vi "振动demo.vi"() -> ()   [LabVIEW 2020]
uses:
  Database/Global2.vi
  Global_Variable/Global.vi
  Global_Variable/Global1.vi
  Global_Variable/A131258.vi
  <vilib>/addons/database/Connection.llb/DB Tools Open Connec (String).vi
  <vilib>/addons/database/Connection.llb/Conn Execute.vi
  <vilib>/addons/database/Recordset.llb/Rec Fetch Recordset Data (R).vi
  <vilib>/Utility/config.llb/NI_LVConfig.lvlib
  <vilib>/addons/database/NI_Database_API.lvlib
panel:
  out "result":string
  out "FdeviceID":string
  out "deviceID":string
  out "USERID":string
  out "productID":string
  out "CODEID":string
  in  "附加信息":string
  in  "设备状态":enum16{"设备离线", "设备正常", "设备缺料", "设备故障", "质量报警"}(ring)=enum."设备故障"
  in  "附加信息 2":string
  in  "设备状态 2":enum16{"设备离线", "设备正常", "设备缺料", "设备故障", "质量报警"}(ring)=enum."设备缺料"
  in  "附加信息 3":string
  in  "设备状态 3":enum16{"设备离线", "设备正常", "设备缺料", "设备故障", "质量报警"}(ring)=enum."质量报警"
  out "产品型号":string
  out "联机模式":string
  out "用户权限":string
  out "用户名":string
  in  "判定结果1":bool[][](array[boolean])=[[TRUE]]
  in  "选项卡控件 2":enum32{"主页面", "参数设置"}(tab)
  out "产品条码":string
  out "判定结果":bool
  out "振动NHV-FFT":cluster{"f0":dbl, "df":dbl, "magnitude":dbl[]}[](graph)
  out "振动NVH-Order":cluster{"f0":dbl, "df":dbl, "magnitude":dbl[]}[](graph)
  in  "表格控件":string[][](table)
  in  "设备故障":bool
  in  "设备缺料":bool
  in  "质量报警":bool
  out "上序结果":bool
  out "字符串":string
  in  "请输入添加的产品名称":string
  in  "请选择要删除的产品":string(combo)
  in  "振动判定范围":T1={"频率检测段1范围"={"单位"="Hz", "下限"=0.0, "上限"=100.0}, "频率检测段2范围"={"单位"="Hz", "下限"=100.0, "上限"=1000.0}, "频率检测段3范围"={"单位"="Hz", "下限"=1000.0, "上限"=2000.0}, "频率检测段4范围"={"单位"="Hz", "下限"=2000.0, "上限"=3000.0}, "频率检测段5范围"={"单位"="Hz", "下限"=3000.0, "上限"=10000.0}}
  in  "振动判定":T2={"频率检测段1振幅"={"单位"="dB", "下限"=0.0, "上限"=50.0}, "频率检测段2振幅"={"单位"="dB", "下限"=0.0, "上限"=40.0}, "频率检测段3振幅"={"单位"="dB", "下限"=0.0, "上限"=40.0}, "频率检测段4振幅"={"单位"="dB", "下限"=0.0, "上限"=40.0}, "频率检测段5振幅"={"单位"="dB", "下限"=0.0, "上限"=40.0}}
  in  "产品型号":string(combo)
  in  "删除":bool
  in  "确定":bool
  in  "添加":bool
  in  "退出":bool
  in  "更新":bool
  in  "确定按钮":bool
  # "060芯轴总成NVH评价"
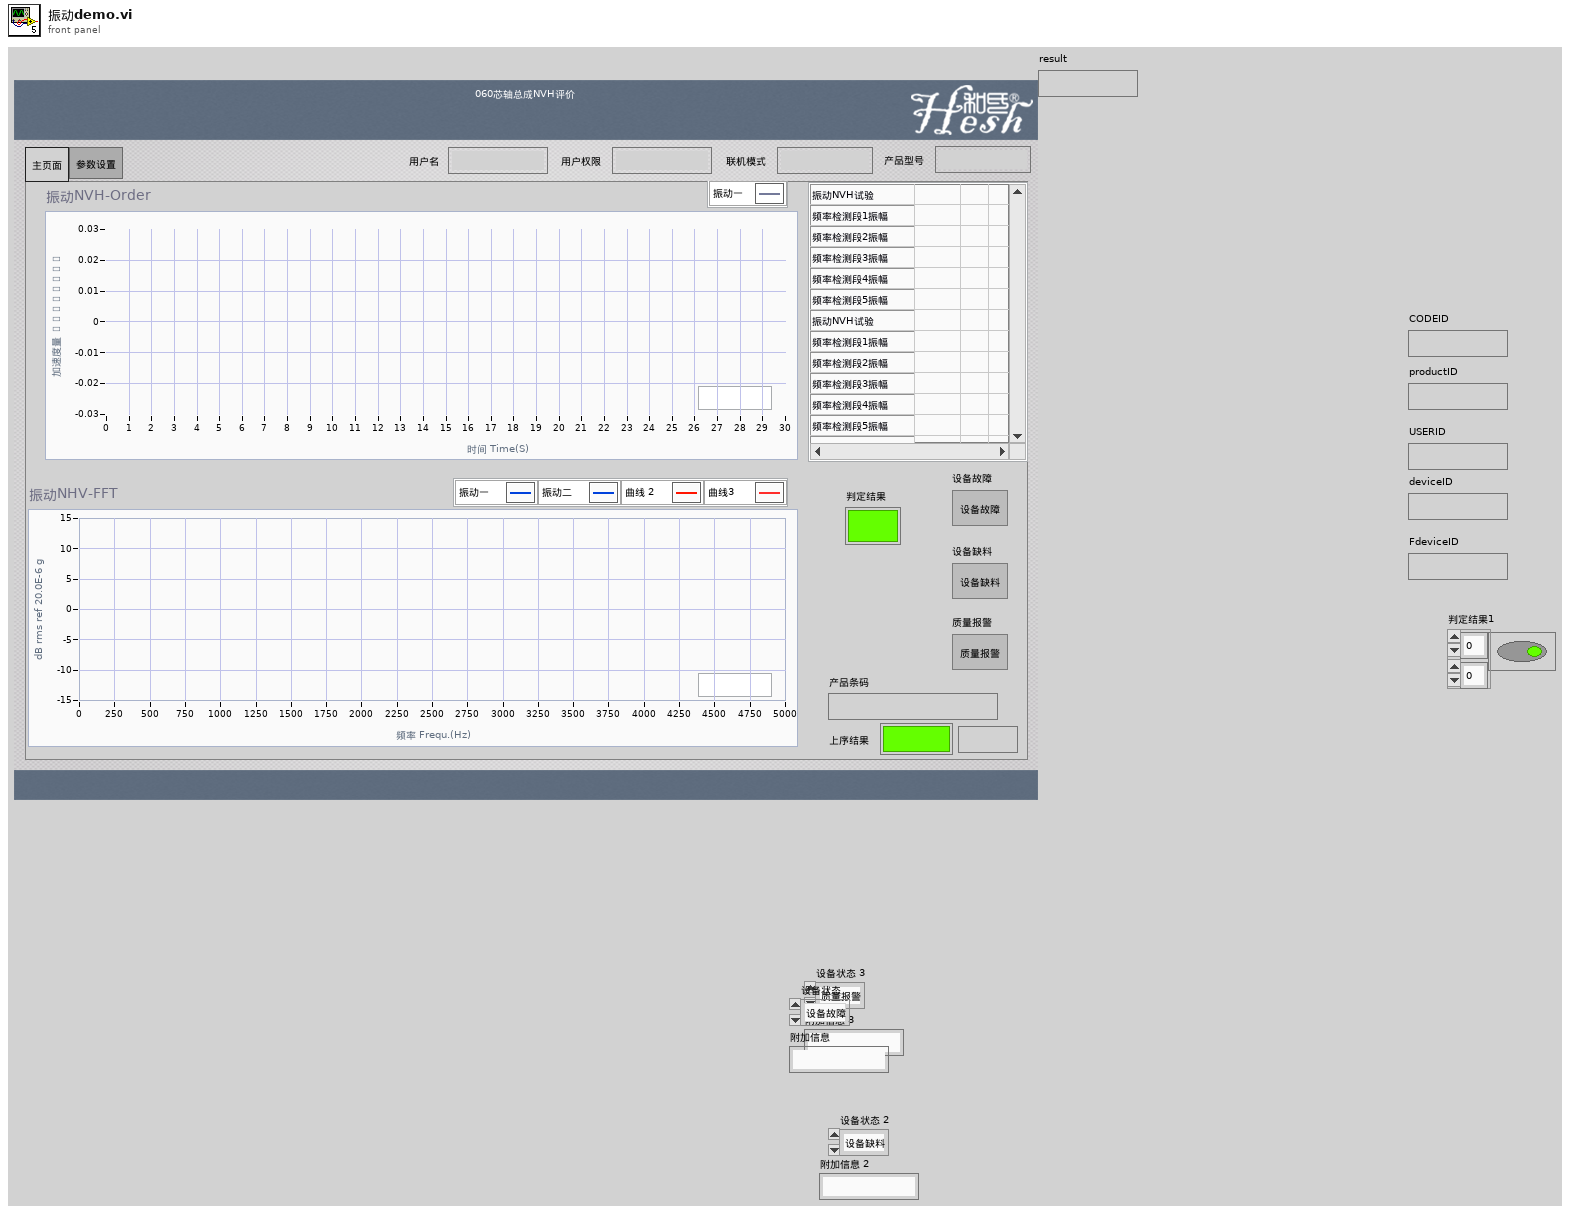
[diagram p1: front panel]
types:
  T1 = cluster{"频率检测段1范围":cluster{"单位":string, "下限":dbl, "上限":dbl}, "频率检测段2范围":cluster{"单位":string, "下限":dbl, "上限":dbl}, "频率检测段3范围":cluster{"单位":string, "下限":dbl, "上限":dbl}, "频率检测段4范围":cluster{"单位":string, "下限":dbl, "上限":dbl}, "频率检测段5范围":cluster{"单位":string, "下限":dbl, "上限":dbl}}
  T2 = cluster{"频率检测段1振幅":cluster{"单位":string, "下限":dbl, "上限":dbl}, "频率检测段2振幅":cluster{"单位":string, "下限":dbl, "上限":dbl}, "频率检测段3振幅":cluster{"单位":string, "下限":dbl, "上限":dbl}, "频率检测段4振幅":cluster{"单位":string, "下限":dbl, "上限":dbl}, "频率检测段5振幅":cluster{"单位":string, "下限":dbl, "上限":dbl}}
  T3 = cluster{"设备名称":string, "操作人员":string, "设备状态":enum16{"设备离线", "设备正常", "设备缺料", "设备故障", "质量报警"}, "附加信息":string}
  T4 = enum32{"Invalid", "Standard", "Closed", "Hidden", "Minimized", "Maximized"}
  T5 = cluster{"用户编号":string, "用户名":string, "用户密码(密文)":string, "用户权限":string}
  T6 = typedef "svc_Spectrum Info.ctl" = cluster{"channel name":string, "description":string, "x-axis units":T7, "spectral info":cluster{"spectrum type":T8, "linear/dB":enum16{"linear", "dB"}, "window":u16, "window size":i32, "FFT size":i32}, "engineering units":T9, "custom label":string, "dB reference [EU]":dbl, "peak units":enum16{"rms", "peak", "peak-peak"}, "weighting filter":T10, "spectral density?":bool, "unit label":string, "spectrum skewed?":bool, "complimentary spectrum units":T11}
  T7 = typedef "svc_X-Axis Units.ctl" = u16
  T8 = typedef "svc_Spectrum Type.ctl" = enum16{"FFT Spectrum [complex]", "Amplitude [Magnitude]", "Power [Magnitude^2]", "Cross Spectrum [complex]", "Frequency Response [Complex]"}
  T9 = typedef "svc_Engineering Units Text Ring.ctl" = u16
  T10 = typedef "svc_Weighting Filter Text Ring.ctl" = u16
  T11 = typedef "svc_Complimentary Spectrum Units.ctl" = enum16{"none", "radians", "degrees", "cycles", "imaginary"}
  T12 = cluster{i64, i64, i64, "result":string, "result string":string}
  T13 = cluster{i64, i64, i64, "result":string, "result string":string}[]
  T14 = typedef "NI_Database_API.lvlib/Conn ObjectReference.ctl" = refnum<k1>
  T15 = cluster{i64, i64, "condition":string, dbl, "下限":dbl, "上限":dbl, string, string}
  T16 = cluster{i64, i64, "condition":string, dbl, "下限":dbl, "上限":dbl, string, string}[]
  T17 = cluster{i64, i64, dbl, "下限":dbl, "上限":dbl, string, string}
  T18 = typedef "NI_Database_API.lvlib/Rec ObjectReference.ctl" = refnum<k1>
  T19 = typedef "NI_LVConfig.lvlib/Config Data RefNum.ctl" = refnum<k1>
  T20 = cluster{"设备名称":string, "用户名":string, "设备状态":enum16{"设备离线", "设备正常", "设备缺料", "设备故障", "质量报警"}, "附加信息":string}
  T21 = cluster{"设备名称":string, "用户名":string, "设备状态 2":enum16{"设备离线", "设备正常", "设备缺料", "设备故障", "质量报警"}, "附加信息 2":string}
  T22 = cluster{"设备名称":string, "用户名":string, "设备状态 3":enum16{"设备离线", "设备正常", "设备缺料", "设备故障", "质量报警"}, "附加信息 3":string}
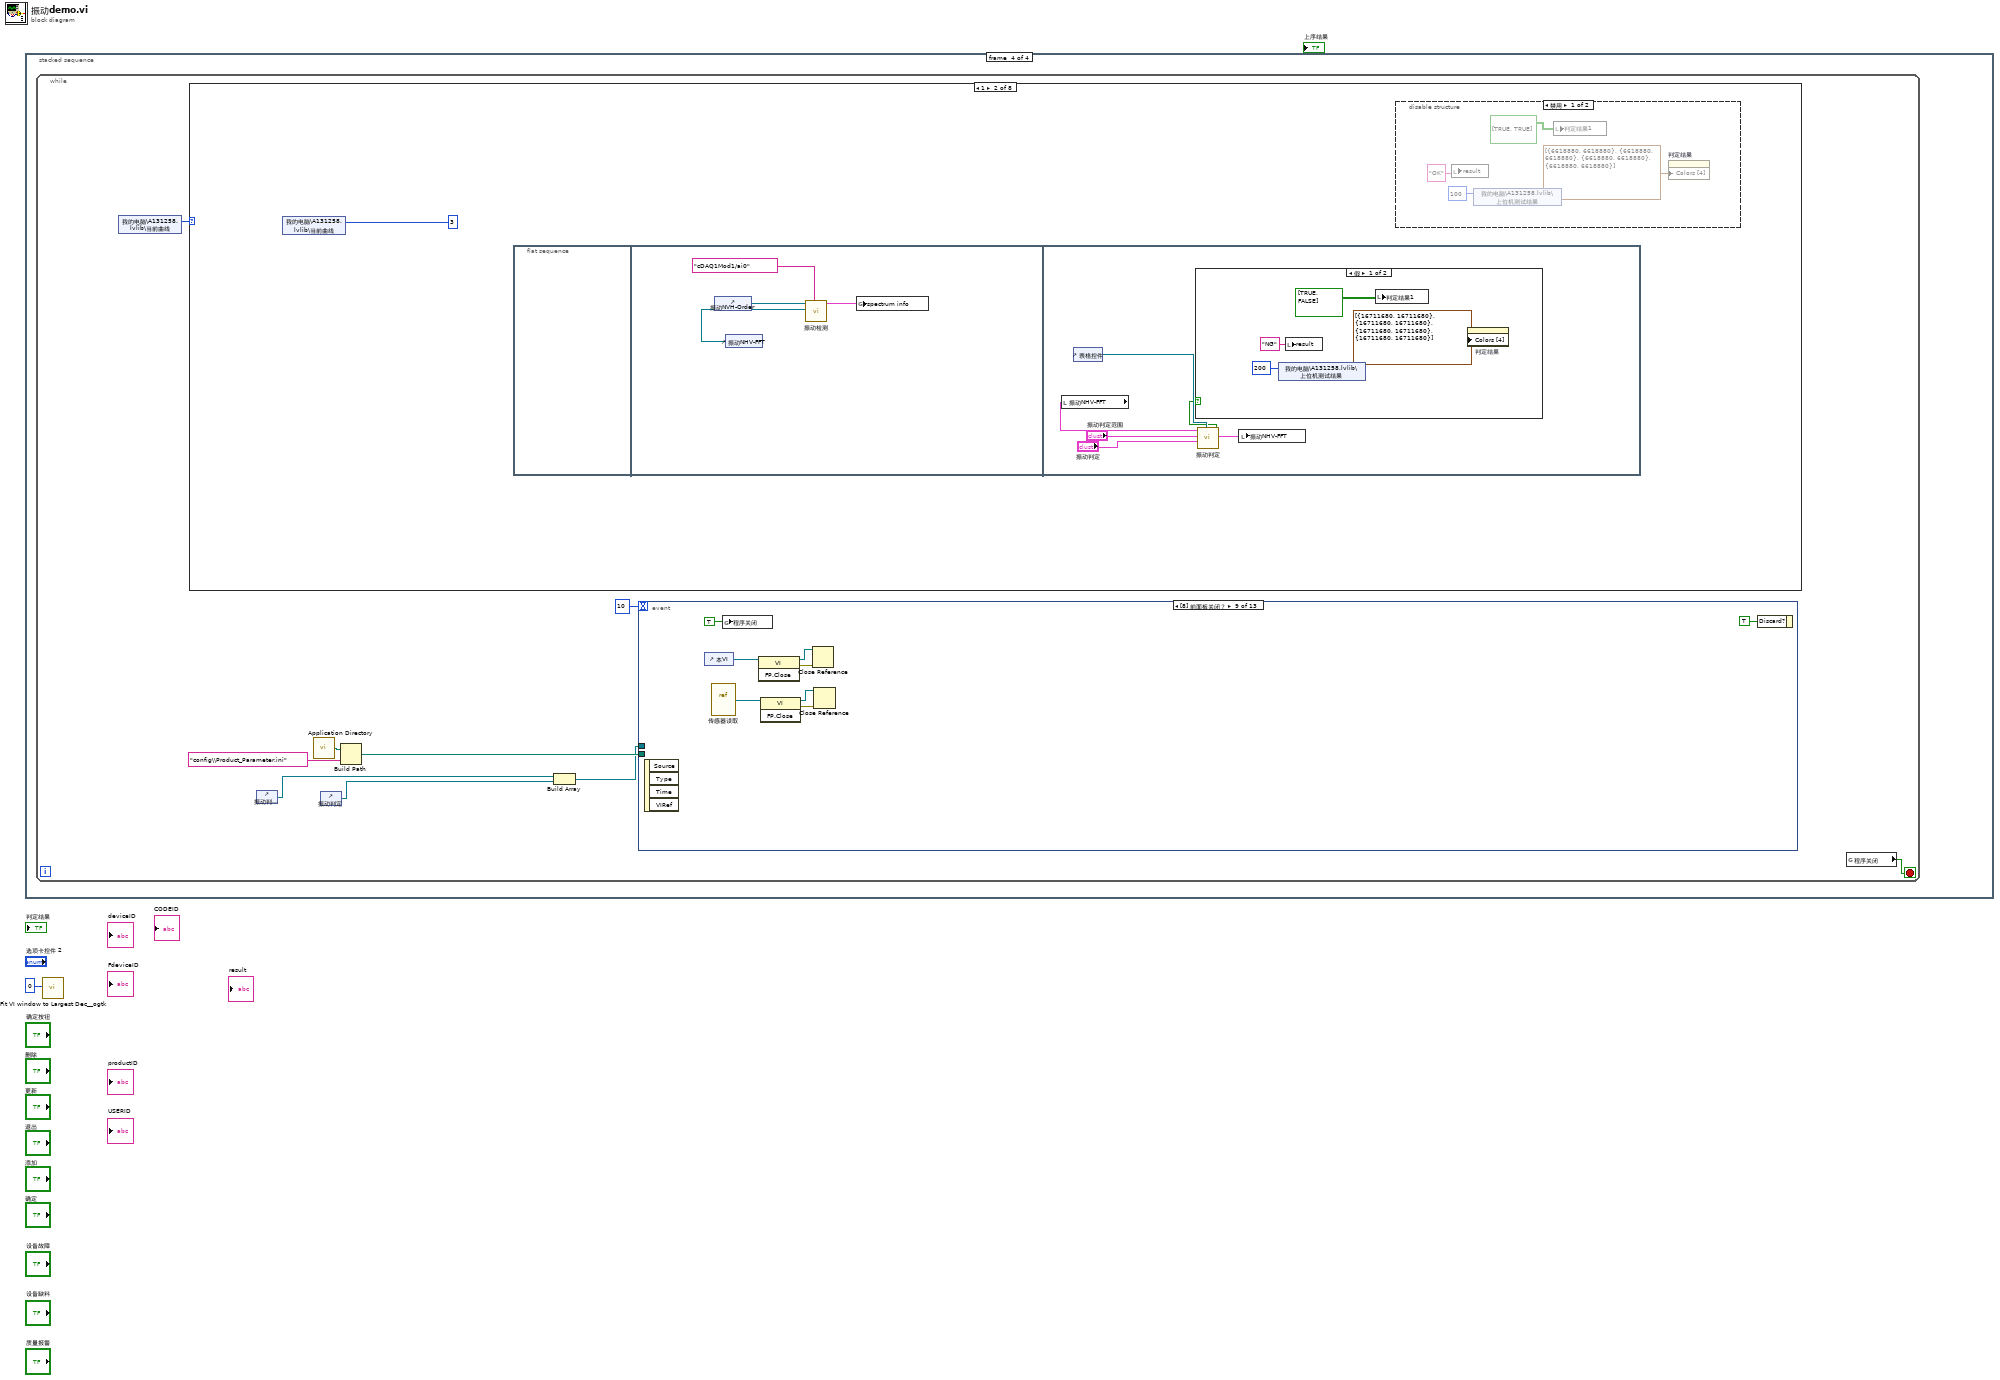
[diagram p0: block diagram]
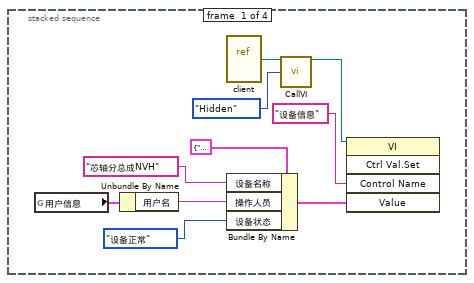
[diagram p2: hidden frame]
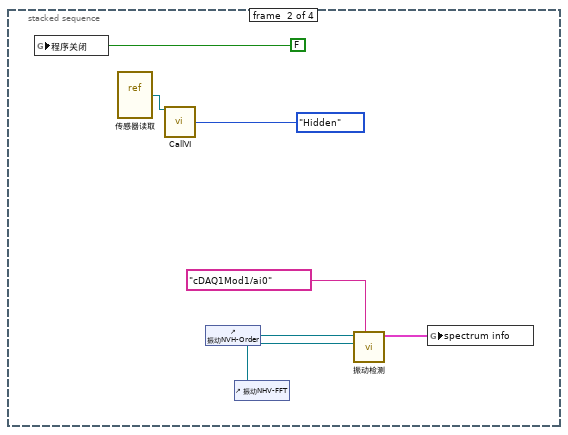
[diagram p3: hidden frame]
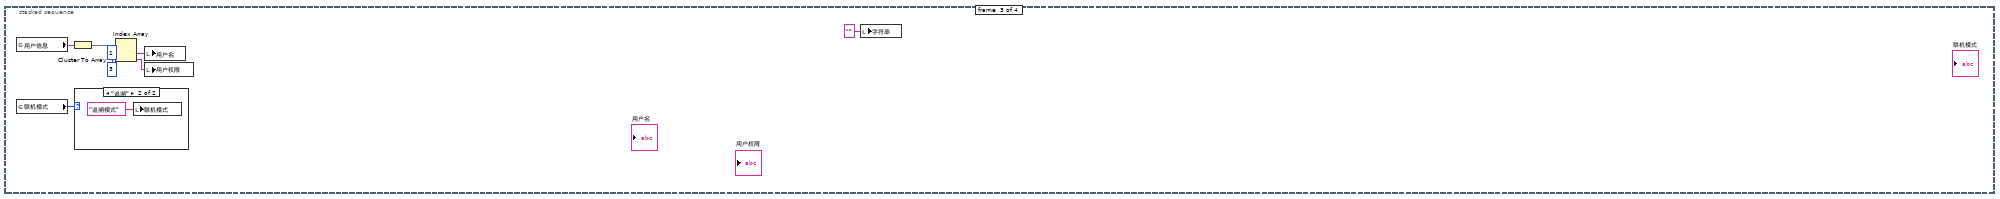
[diagram p4: hidden frame]
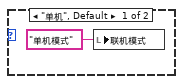
[diagram p5: hidden frame]
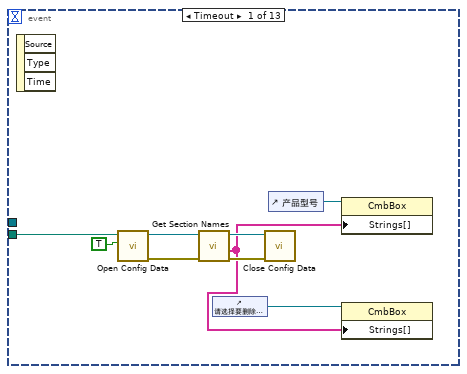
[diagram p6: hidden frame]
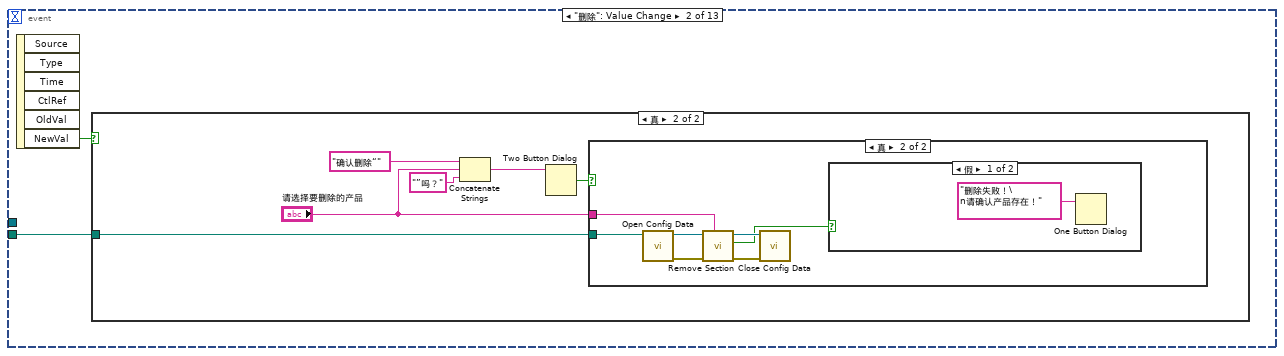
[diagram p7: hidden frame]
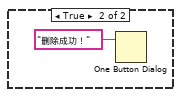
[diagram p10: hidden frame]
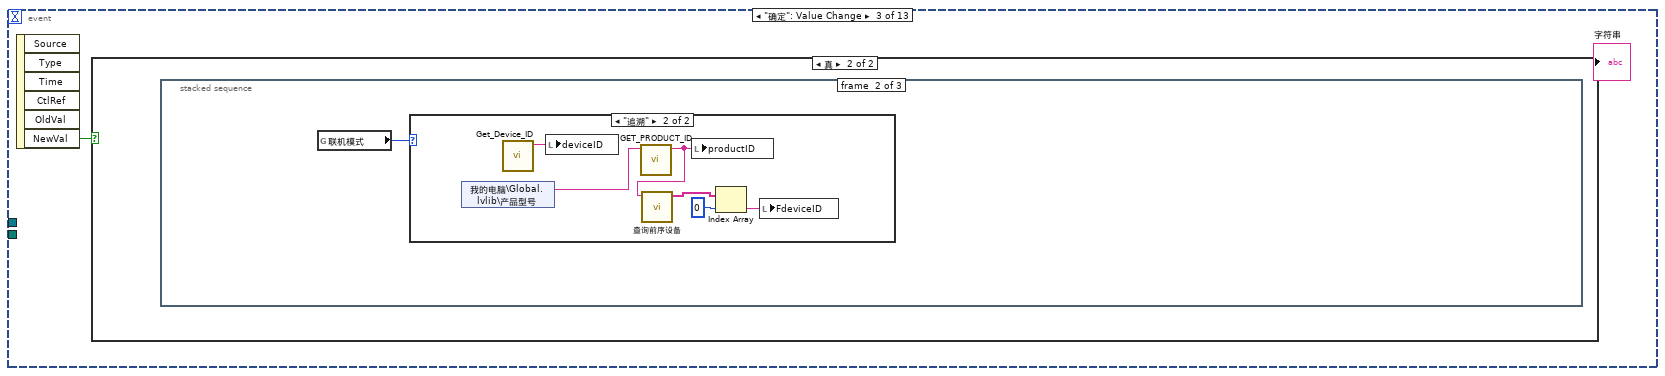
[diagram p11: hidden frame]
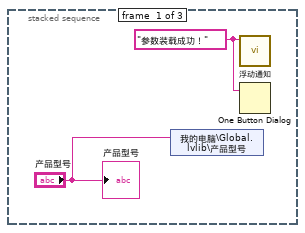
[diagram p13: hidden frame]
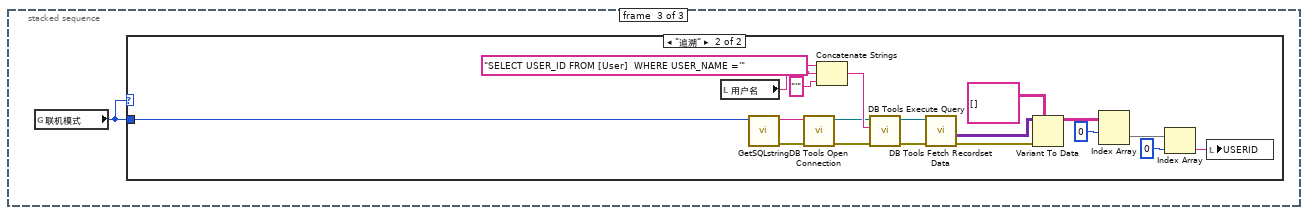
[diagram p15: hidden frame]
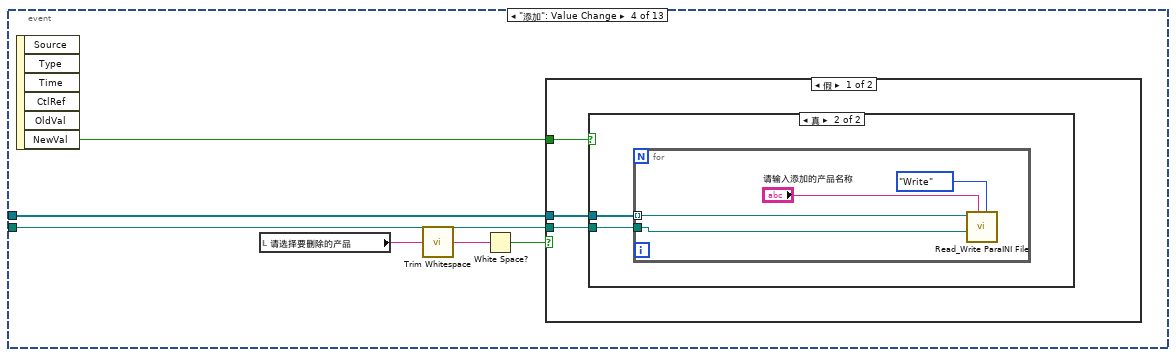
[diagram p17: hidden frame]
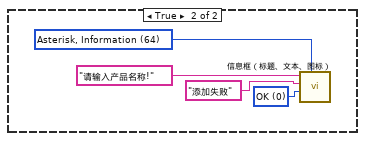
[diagram p19: hidden frame]
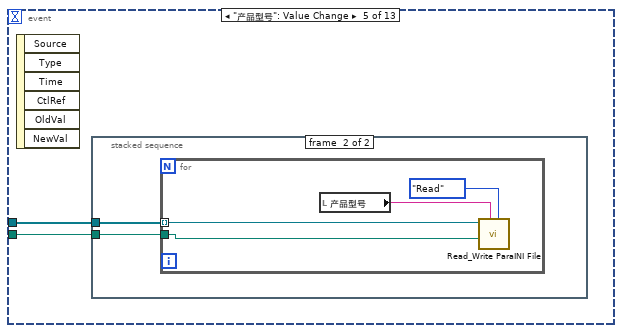
[diagram p20: hidden frame]
diagram:
  n1 = stacked-sequence {
    frame #0 {
      n2 = global read "Global2.vi" "用户信息"() -> (w11:T5)
      n3 = Unbundle By Name(w11) -> ("用户名"=w10:string)
      n4 = vi-ref "client.vi"() -> (w8:refnum<vi>)
      n5 = Bundle By Name(cluster=T3 {"设备名称"="", "操作人员"="", "设备状态"=enum."设备正常", "附加信息"=""} ("设备信息"), "设备名称"="芯轴分总成NVH", "操作人员"=w10, "设备状态"=enum16{"设备离线", "设备正常", "设备缺料", "设备故障", "质量报警"}."设备正常") -> (w9:T3)
      n6 = call "CallVI.vi"("VI引用"=w8, "状态"=T4."Hidden") -> ("VI引用输出"=w7:refnum<vi>)  [unwired: 11 in, 2 out]
      n7 = invoke class="VI" method="Ctrl Val.Set"(reference=w7, "Control Name"="设备信息" ("控件名"), "Value"=w9) -> ()  [unwired: 2 in, 5 out]
    }
    frame #1 {
      n8 = global write "Global.vi" "程序关闭"(FALSE ("程序关闭")) -> ()
      n9 = vi-ref "传感器读取.vi"() -> (w17:refnum<vi>)
      n10 = call "CallVI.vi"("VI引用"=w17, "状态"=T4."Hidden") -> ()  [unwired: 11 in, 3 out]
      n11 = control-ref of="振动NVH-Order"() -> (w15:refnum<vi>)
      n12 = control-ref of="振动NHV-FFT"() -> (w14:refnum<vi>)
      n13 = call "振动检测.vi"("通道输入"=tag "cDAQ1Mod1/ai0" ("DAQmx物理通道"), "WFGraph引用句柄FFT"=w14, "WFGraph引用句柄Order"=w15) -> ("spectrum info"=w13:T6[])  [unwired: 7 in, 1 out]
      n14 = global write "Global1.vi" "spectrum info"(w13) -> ()
    }
    frame #2 {
      n15 = global read "Global2.vi" "用户信息"() -> (w26:T5)
      n16 = global read "Global2.vi" "联机模式"() -> (w20:enum16{"单机", "追溯"})
      n17 = Cluster To Array(cluster=w26) -> (array=w25:string[])
      n18 = case shown="\"追溯\"" w20 {
        frame "单机", Default {
          n19 = local write "联机模式"("单机模式" ("联机模式")) -> ()
        }
        frame "追溯" {
          n20 = local write "联机模式"("追溯模式" ("联机模式")) -> ()
        }
      }
      n21 = Index Array(array=w25, index #1=1 ("索引"), index #2=3 ("索引")) -> (element #1=w22:string, element #2=w21:string)
      n22 = local write "用户名"(w22) -> ()
      n23 = local write "用户权限"(w21) -> ()
      n24 = local write "字符串"("" ("字符串")) -> ()
    }
    frame #3 {
      n25 = while {
        stop <- w29 stop-if-true
        n26 = shared-variable "我的电脑\\A131258.lvlib\\当前曲线"() -> (w37:i16)  [unwired: 1 in, 1 out]
        n27 = case shown="1" w37 {
          frame 0, Default {
          }
          frame 1 {
            n28 = shared-variable "我的电脑\\A131258.lvlib\\当前曲线"(i16 3 ("当前曲线")) -> ()  [unwired: 1 in, 1 out]
            n29 = flat-sequence {
              frame #0 {
              }
              frame #1 {
                n30 = control-ref of="振动NVH-Order"() -> (w194:refnum<vi>)
                n31 = control-ref of="振动NHV-FFT"() -> (w193:refnum<vi>)
                n32 = call "振动检测.vi"("通道输入"=tag "cDAQ1Mod1/ai0" ("DAQmx物理通道"), "WFGraph引用句柄FFT"=w193, "WFGraph引用句柄Order"=w194) -> ("spectrum info"=w191:T6[])  [unwired: 7 in, 1 out]
                n33 = global write "Global1.vi" "spectrum info"(w191) -> ()
              }
              frame #2 {
                n34 = local read "振动NHV-FFT"() -> (w200:cluster{"f0":dbl, "df":dbl, "magnitude":dbl[]}[])
                n35 = control-ref of="表格控件"() -> (w196:refnum<vi>)
                n36 = call "振动判定.vi"("Result"=w196, "振动判定"="振动判定", "振动判定范围"="振动判定范围", "FFT"=w200) -> ("FFT 2"=w197:cluster{"f0":dbl, "df":dbl, "magnitude":dbl[]}[], "OK？"=w195:bool)  [unwired: 6 in]
                n37 = case shown="假" w195 {
                  frame False {
                    n38 = shared-variable "我的电脑\\A131258.lvlib\\上位机测试结果"(i16 200 ("当前曲线")) -> ()  [unwired: 1 in, 1 out]
                    n39 = local write "result"("NG" ("result")) -> ()
                    n40 = local write "判定结果1"(bool[][] [[TRUE, FALSE]] ("判定结果1")) -> ()
                    n41 = property on="判定结果" class="Bool (严格)"("Colors [4]"=cluster{u32, u32}[] [{16711680, 16711680}, {16711680, 16711680}, {16711680, 16711680}, {16711680, 16711680}]) -> ()  [unwired: 2 in, 2 out]
                  }
                  frame True {
                    n42 = local write "result"("OK" ("result")) -> ()
                    n43 = shared-variable "我的电脑\\A131258.lvlib\\上位机测试结果"(i16 100 ("当前曲线")) -> ()  [unwired: 1 in, 1 out]
                    n44 = local write "判定结果1"(bool[][] [[TRUE, TRUE]] ("判定结果1")) -> ()
                    n45 = property on="判定结果" class="Bool (严格)"("Colors [4]"=cluster{u32, u32}[] [{6618880, 6618880}, {6618880, 6618880}, {6618880, 6618880}, {6618880, 6618880}]) -> ()  [unwired: 2 in, 2 out]
                  }
                }
                n46 = local write "振动NHV-FFT"(w197) -> ()
              }
            }
            n47 = disable-structure shown="禁用" {
              frame Disabled {
                n48 = local write "result"("OK" ("result")) -> ()
                n49 = shared-variable "我的电脑\\A131258.lvlib\\上位机测试结果"(i16 100 ("当前曲线")) -> ()  [unwired: 1 in, 1 out]
                n50 = local write "判定结果1"(bool[][] [[TRUE, TRUE]] ("判定结果1")) -> ()
                n51 = property on="判定结果" class="Bool (严格)"("Colors [4]"=cluster{u32, u32}[] [{6618880, 6618880}, {6618880, 6618880}, {6618880, 6618880}, {6618880, 6618880}]) -> ()  [unwired: 2 in, 2 out]
              }
              frame Enabled {
              }
            }
          }
          frame 2 {
            n52 = for {
              N: 6 -> [_]
              tunnel: [cluster{"f0":dbl, "df":dbl, "magnitude":dbl[]} {"f0"=0.0, "df"=0.0, "magnitude"=[]} ("power spectrum [dB EU]")] -> w212 mode=indexing
            }
            "振动NVH-Order" <- w212
            "振动NHV-FFT" <- w212
            n53 = property on="表格控件" class="Tbl (严格)"("Value"=string[][] [] ("表格控件"), "Row Headers[]"=string[] [] ("行首字符串[]")) -> ()  [unwired: 2 in, 2 out]
          }
          frame 3 {
            n54 = control-ref of="表格控件"() -> (w215:refnum<vi>)
            n55 = shared-variable "我的电脑\\A131258.lvlib\\当前曲线"(i16 4 ("当前曲线")) -> ()  [unwired: 1 in, 1 out]
            n56 = Wait (ms)(milliseconds to wait=u32 200 ("等待时间（毫秒）")) -> ()  [unwired: 1 out]
            n57 = control-ref of="振动NHV-FFT"() -> (w216:refnum<vi>)
            n58 = global write "Global.vi" "Result"(w215) -> ()
            n59 = control-ref of="振动NVH-Order"() -> (w214:refnum<vi>)
            n60 = global write "A131258.vi" "加速度"(w216) -> ()
            n61 = call "浮动通知.vi"("通知内容"="报表生成中") -> ()  [unwired: 11 in]
            n62 = global write "A131258.vi" "频率"(w214) -> ()
          }
          frame 4 {
            n63 = stacked-sequence {
              frame #0 {
                n64 = local read "产品条码"() -> (w220:string)
                n65 = call "Report_A131258.vi"("文件重命名"=TRUE, "文件名称"=w220, "布尔数组"="判定结果1") -> ()  [unwired: 8 in, 1 out]
              }
              frame #1 {
                n66 = global read "Global2.vi" "联机模式"() -> (w223:enum16{"单机", "追溯"})
                n67 = case shown="\"追溯\"" w223 {
                  frame "单机", Default {
                  }
                  frame "追溯" {
                    n68 = local read "result"() -> (w224:string)
                    n69 = local read "USERID"() -> (w250:string)
                    n70 = Decimal String To Number(string=w250, default (0L)=i64 0 ("默认(0 I32)")) -> (number=w251:i64)  [unwired: 1 in, 1 out]
                    n71 = local read "deviceID"() -> (w242:string)
                    n72 = global read "Global2.vi" "联机模式"() -> (w225:enum16{"单机", "追溯"})
                    n73 = local read "CODEID"() -> (w244:string)
                    n74 = Get Date/Time String(date format (0)=enum16{"short", "long", "abbreviated"}."short" ("日期格式(0)"), want seconds? (F)=FALSE ("需要秒？(F)")) -> (date string=w246:string, time string=w247:string)  [unwired: 1 in]
                    n75 = Decimal String To Number(string=w242, default (0L)=i64 0 ("默认(0 I32)")) -> (number=w243:i64)  [unwired: 1 in, 1 out]
                    n76 = Concatenate Strings(w246, " " ("字符串"), w247) -> (w249:string)
                    n77 = Decimal String To Number(string=w244, default (0L)=i64 0 ("默认(0 I32)")) -> (number=w245:i64)  [unwired: 1 in, 1 out]
                    n78 = Search and Replace String(replace all?=TRUE ("替换全部？(F)"), input string=w249, search string="/" ("替换字符串(\"\")"), replace string="-" ("替换字符串(\"\")")) -> (result string=w248:string)  [unwired: 4 in, 3 out]
                    n79 = Bundle(w243, w251, w245, "result"=w224, "result string"=w248) -> (w240:T12)  [unwired: 1 in]
                    n80 = call "GetSQLstring.vi"("联机模式"=w225) -> ("错误输出"=w237:errorcluster, "连接字符串"=w236:string)  [unwired: 9 in]
                    n81 = Build Array(w240) -> (w241:T13)
                    n82 = call-poly <vilib>:"DB Tools Open Connection.vi"("error in (no error)"=w237, "connection information"=w236) -> ("error out"=w235:errorcluster, "connection reference"=w238:T14)  [unwired: 6 in]
                    n83 = for {
                      tunnel: w241 -> [w256] mode=indexing
                      tunnel: w238 -> [w254]
                      shift-right: [w252] -> w239
                      shift-left: w235 -> [w259]
                      w255 = string[] ["DEVICE_ID", "USER_ID", "CODE_ID", "RESULT_VALUE", "RESULT_TIME"] ("columns")
                      w257 = "Result" ("table")
                      n84 = call <vilib>:"DB Tools Insert Data.vi"("data"=w256, "error in (no error)"=w259, "columns"=w255, "table"=w257, "connection reference"=w254) -> ("error out"=w258:errorcluster, "connection reference out"=w253:T14)  [unwired: 5 in]
                      n85 = case shown="错误" w258 {
                        selector: w258 -> [w260 w281]
                        tunnel: w255 -> [_ w278]
                        tunnel: w253 -> [w261 w270]
                        tunnel: w257 -> [_ w282]
                        tunnel: w256 -> [_ w274]
                        tunnel: [w261 w269] -> _
                        tunnel: [w260 w268] -> w252
                        frame No Error {
                        }
                        frame Error {
                          n86 = Array Subset(array=w278, index=3 ("长度"), length=2 ("长度")) -> (w279:string[])
                          n87 = Unbundle(w274) -> (w263:i64, w266:i64, "result"=w273:string, "result string"=w272:string)  [unwired: 1 out]
                          n88 = Bundle("result"=w273, "result string"=w272) -> (w271:cluster{"result":string, "result string":string})  [unwired: 1 in]
                          n89 = Number To Decimal String(number=w266) -> (decimal integer string=w267:string)  [unwired: 1 in]
                          n90 = Number To Decimal String(number=w263) -> (decimal integer string=w262:string)  [unwired: 1 in]
                          n91 = call <vilib>:"Clear Errors.vi"("error in (no error)"=w281) -> ("error out"=w280:errorcluster)  [unwired: 5 in, 1 out]
                          n92 = Concatenate Strings("WHERE CODE_ID =" ("condition"), w267, "AND DEVICE_ID = ", w262) -> (w275:string)
                          n93 = call <vilib>:"DB Tools Update Data.vi"("condition"=w275, "data"=w271, "error in (no error)"=w280, "columns"=w279, "table"=w282, "connection reference"=w270) -> ("error out"=w268:errorcluster, "connection reference out"=w269:T14)  [unwired: 4 in]
                        }
                      }
                    }
                    n94 = call <vilib>:"Simple Error Handler.vi"("error in (no error)"=w239) -> ()  [unwired: 4 in, 5 out]
                  }
                }
              }
              frame #2 {
                n95 = global read "Global2.vi" "联机模式"() -> (w283:enum16{"单机", "追溯"})
                n96 = case shown="\"追溯\"" w283 {
                  tunnel: w283 -> [_ w286]
                  frame "单机", Default {
                  }
                  frame "追溯" {
                    w285 = -999.9 ("下限")
                    w342 = 2 ("索引 (行)")
                    w343 = 1 ("索引 (行)")
                    w344 = 0 ("索引 (行)")
                    n97 = control-ref of="表格控件"() -> (w352:refnum<vi>)
                    n98 = local read "振动判定"() -> (w336:T2)
                    n99 = property class="Tbl (严格)"(reference=w352) -> ("Value"=w351:string[][])  [unwired: 1 in, 2 out]
                    n100 = Unbundle(w336) -> ("频率检测段1振幅"=w337:cluster{"单位":string, "下限":dbl, "上限":dbl}, "频率检测段2振幅"=w335:cluster{"单位":string, "下限":dbl, "上限":dbl}, "频率检测段3振幅"=w334:cluster{"单位":string, "下限":dbl, "上限":dbl}, "频率检测段4振幅"=w333:cluster{"单位":string, "下限":dbl, "上限":dbl}, "频率检测段5振幅"=w332:cluster{"单位":string, "下限":dbl, "上限":dbl})
                    n101 = local read "deviceID"() -> (w320:string)
                    n102 = local read "CODEID"() -> (w318:string)
                    n103 = Index Array(array=w351, index (row) #1=1 ("索引 (行)"), index (row) #2=2 ("索引 (行)"), index (row) #3=3 ("禁用的索引 (列)"), index (row) #4=4 ("索引 (列)"), index (row) #5=5 ("索引 (行)")) -> (element #1=w345:string[], element #2=w341:string[], element #3=w340:string[], element #4=w339:string[], element #5=w338:string[])  [unwired: 5 in]
                    n104 = Unbundle(w337) -> ("上限"=w291:dbl)  [unwired: 2 out]
                    n105 = Unbundle(w335) -> ("上限"=w290:dbl)  [unwired: 2 out]
                    n106 = Unbundle(w332) -> ("上限"=w287:dbl)  [unwired: 2 out]
                    n107 = Unbundle(w334) -> ("上限"=w289:dbl)  [unwired: 2 out]
                    n108 = Unbundle(w333) -> ("上限"=w288:dbl)  [unwired: 2 out]
                    n109 = Decimal String To Number(string=w318, default (0L)=i64 0 ("长度")) -> (number=w316:i64)  [unwired: 1 in, 1 out]
                    n110 = Index Array(array=w340, index #1=w344, index #2=w343, index #3=w342) -> (element #1=w308:string, element #2=w299:string, element #3=w294:string)
                    n111 = Index Array(array=w345, index #1=w344, index #2=w343, index #3=w342) -> (element #1=w310:string, element #2=w301:string, element #3=w296:string)
                    n112 = Index Array(array=w341, index #1=w344, index #2=w343, index #3=w342) -> (element #1=w309:string, element #2=w300:string, element #3=w295:string)
                    n113 = Index Array(array=w338, index #1=w344, index #2=w343, index #3=w342) -> (element #1=w306:string, element #2=w297:string, element #3=w292:string)
                    n114 = Index Array(array=w339, index #1=w344, index #2=w343, index #3=w342) -> (element #1=w307:string, element #2=w298:string, element #3=w293:string)
                    n115 = Decimal String To Number(string=w320, default (0L)=i64 0 ("长度")) -> (number=w317:i64)  [unwired: 1 in, 1 out]
                    n116 = Fract/Exp String To Number(string=w307) -> (number=w303:dbl)  [unwired: 3 in, 1 out]
                    n117 = Fract/Exp String To Number(string=w306) -> (number=w302:dbl)  [unwired: 3 in, 1 out]
                    n118 = Fract/Exp String To Number(string=w308) -> (number=w304:dbl)  [unwired: 3 in, 1 out]
                    n119 = Fract/Exp String To Number(string=w309) -> (number=w305:dbl)  [unwired: 3 in, 1 out]
                    n120 = Fract/Exp String To Number(string=w310) -> (number=w311:dbl)  [unwired: 3 in, 1 out]
                    n121 = Bundle(w317, w316, "condition"="检测段1振幅", w311, "下限"=w285, "上限"=w291, w301, w296) -> (w327:T15)  [unwired: 1 in]
                    n122 = Bundle(w317, w316, "condition"="检测段2振幅", w305, "下限"=w285, "上限"=w290, w300, w295) -> (w326:T15)  [unwired: 1 in]
                    n123 = Bundle(w317, w316, "condition"="检测段3振幅", w304, "下限"=w285, "上限"=w289, w299, w294) -> (w324:T15)  [unwired: 1 in]
                    n124 = Bundle(w317, w316, "condition"="检测段4振幅", w303, "下限"=w285, "上限"=w288, w298, w293) -> (w323:T15)  [unwired: 1 in]
                    n125 = Bundle(w317, w316, "condition"="检测段5振幅", w302, "下限"=w285, "上限"=w287, w297, w292) -> (w322:T15)  [unwired: 1 in]
                    n126 = call "GetSQLstring.vi"("联机模式"=w286) -> ("错误输出"=w329:errorcluster, "连接字符串"=w330:string)  [unwired: 9 in]
                    n127 = Build Array(w327, w326, w324, w323, w322) -> (w325:T16)
                    n128 = call-poly <vilib>:"DB Tools Open Connection.vi"("error in (no error)"=w329, "connection information"=w330) -> ("error out"=w331:errorcluster, "connection reference"=w328:T14)  [unwired: 6 in]
                    n129 = for {
                      tunnel: w325 -> [w357] mode=indexing
                      tunnel: w328 -> [w355]
                      shift-right: [w353] -> _
                      shift-left: w331 -> [w360]
                      w356 = string[] ["DEVICE_ID", "CODE_ID", "TEST_NAME", "TEST_VALUE", "TEST_VALUE_MIN", "TEST_VALUE_MAX", "TEST_VALUE_UNIT", "TEST_VALUE_RESULT"] ("columns")
                      w358 = "Test" ("table")
                      n130 = call <vilib>:"DB Tools Insert Data.vi"("data"=w357, "error in (no error)"=w360, "columns"=w356, "table"=w358, "connection reference"=w355) -> ("error out"=w359:errorcluster, "connection reference out"=w354:T14)  [unwired: 5 in]
                      n131 = case shown="错误" w359 {
                        selector: w359 -> [w361 w386]
                        tunnel: w356 -> [_ w383]
                        tunnel: w354 -> [w362 w368]
                        tunnel: w358 -> [_ w387]
                        tunnel: w357 -> [_ w377]
                        tunnel: [w362 w367] -> _
                        tunnel: [w361 w366] -> w353
                        frame No Error {
                        }
                        frame Error {
                          n132 = Delete From Array(array=w383, length=1 ("长度"), index=2 ("索引")) -> (array with subset deleted=w384:string[])  [unwired: 1 out]
                          n133 = Unbundle(w377) -> (w376:i64, w364:i64, "condition"=w369:string, w375:dbl, "下限"=w374:dbl, "上限"=w373:dbl, w372:string, w371:string)
                          n134 = Number To Decimal String(number=w364) -> (decimal integer string=w363:string)  [unwired: 1 in]
                          n135 = Bundle(w376, w364, w375, "下限"=w374, "上限"=w373, w372, w371) -> (w370:T17)  [unwired: 1 in]
                          n136 = call <vilib>:"Clear Errors.vi"("error in (no error)"=w386) -> ("error out"=w385:errorcluster)  [unwired: 5 in, 1 out]
                          n137 = Concatenate Strings("WHERE  TEST_NAME ='" ("condition"), w369, "' ", "AND CODE_ID =" ("condition"), w363) -> (w379:string)
                          n138 = call <vilib>:"DB Tools Update Data.vi"("condition"=w379, "data"=w370, "error in (no error)"=w385, "columns"=w384, "table"=w387, "connection reference"=w368) -> ("error out"=w366:errorcluster, "connection reference out"=w367:T14)  [unwired: 4 in]
                        }
                      }
                    }
                  }
                }
              }
              frame #3 {
                n139 = shared-variable "我的电脑\\A131258.lvlib\\当前曲线"(i16 5 ("当前曲线")) -> ()  [unwired: 1 in, 1 out]
                n140 = local write "字符串"("" ("字符串")) -> ()
              }
            }
          }
          frame 1000 {
            n141 = stacked-sequence {
              frame #0 {
                w392 = "" ("传感器码")
                n142 = shared-variable "我的电脑\\Global.lvlib\\传感器码"(w392) -> ()  [unwired: 1 in, 1 out]
                n143 = local write "产品条码"(w392) -> ()
                n144 = local write "字符串"("" ("传感器码")) -> ()
                n145 = property on="上序结果" class="Bool (严格)"("Colors [4]"=cluster{u32, u32}[] [{12369084, 12369084}, {12369084, 12369084}, {12369084, 12369084}, {12369084, 12369084}]) -> ()  [unwired: 2 in, 2 out]
              }
              frame #1 {
                w395 = "请扫码！" ("通知内容")
                n146 = call "浮动通知.vi"("通知内容"=w395) -> ()  [unwired: 11 in]
                n147 = call "输入框.vi"("提示信息"=w395) -> ("条形码输出"=w394:string)
                "产品条码" <- w394
                n148 = shared-variable "我的电脑\\Global.lvlib\\传感器码"(w394) -> ()  [unwired: 1 in, 1 out]
                n149 = shared-variable "我的电脑\\A131258.lvlib\\当前曲线"(i16 1005 ("当前曲线")) -> ()  [unwired: 1 in, 1 out]
              }
            }
          }
          frame 1005 {
            n150 = local read "产品条码"() -> (w396:string)
            n151 = String Length(string=w396) -> (length=w398:i32)
            n152 = Greater?(x=w398, y=1) -> (0:w399:bool)
            n153 = case shown="真" w399 {
              frame False {
              }
              frame True {
                n154 = shared-variable "我的电脑\\A131258.lvlib\\当前曲线"(i16 1001 ("当前曲线")) -> ()  [unwired: 1 in, 1 out]
              }
            }
          }
          frame 1001 {
            n155 = global read "Global2.vi" "联机模式"() -> (w401:enum16{"单机", "追溯"})
            n156 = case shown="\"追溯\"" w401 {
              frame "单机", Default {
                n157 = shared-variable "我的电脑\\A131258.lvlib\\当前曲线"(i16 1002 ("当前曲线")) -> ()  [unwired: 1 in, 1 out]
              }
              frame "追溯" {
                n158 = stacked-sequence {
                  frame #0 {
                    n159 = local read "产品条码"() -> (w405:string)
                    n160 = local read "productID"() -> (w406:string)
                    n161 = global read "Global2.vi" "联机模式"() -> (w424:enum16{"单机", "追溯"})
                    n162 = call "GetSQLstring.vi"("联机模式"=w424) -> ("错误输出"=w422:errorcluster, "连接字符串"=w423:string)  [unwired: 9 in]
                    n163 = Concatenate Strings("SELECT CODE_ID FROM CODE  WHERE CODE_SENSOR = '" ("字符串"), w405, "'" ("字符串"), " AND PRODUCT_ID= '" ("字符串"), w406, "'" ("字符串")) -> (w421:string)
                    n164 = call-poly <vilib>:"DB Tools Open Connection.vi"("error in (no error)"=w422, "connection information"=w423) -> ("error out"=w415:errorcluster, "connection reference"=w416:T14)  [unwired: 6 in]
                    n165 = call-poly <vilib>:"DB Tools Execute Query.vi"("error in (no error)"=w415, "SQL query"=w421, "connection reference"=w416) -> ("error out"=w419:errorcluster, "recordset reference"=w420:T18)  [unwired: 5 in]
                    n166 = call-poly <vilib>:"DB Tools Fetch Recordset Data.vi"("error in (no error)"=w419, "recordset reference"=w420) -> ("error out"=w412:errorcluster, "recordset data"=w418:variant[][])  [unwired: 3 in, 1 out]
                    n167 = Variant To Data(error in=w412, type=string[][] [], Variant=w418) -> (data=w411:string[][])  [unwired: 1 out]
                    n168 = Index Array(array=w411, index (row)=0 ("索引 (行)")) -> (element=w409:string[])  [unwired: 1 in]
                    n169 = Index Array(array=w409, index=0 ("索引 (行)")) -> (element=w403:string)
                    n170 = local write "CODEID"(w403) -> ()
                    n171 = case shown="\"\"" w403 {
                      frame Default {
                      }
                      frame "" {
                        n172 = shared-variable "我的电脑\\A131258.lvlib\\当前曲线"(i16 0 ("当前曲线")) -> ()  [unwired: 1 in, 1 out]
                        n173 = local write "字符串"("漏序" ("字符串")) -> ()
                        n174 = property on="上序结果" class="Bool (严格)"("Colors [4]"=cluster{u32, u32}[] [{16776704, 16776704}, {16776704, 16776704}, {16776704, 16776704}, {16776704, 16776704}]) -> ()  [unwired: 2 in, 2 out]
                      }
                    }
                  }
                  frame #1 {
                    n175 = local read "CODEID"() -> (w434:string)
                    n176 = local read "FdeviceID"() -> (w429:string)
                    n177 = global read "Global2.vi" "联机模式"() -> (w436:enum16{"单机", "追溯"})
                    n178 = call "GetSQLstring.vi"("联机模式"=w436) -> ("错误输出"=w438:errorcluster, "连接字符串"=w437:string)  [unwired: 9 in]
                    n179 = Concatenate Strings(" SELECT RESULT_VALUE FROM RESULT  WHERE DEVICE_ID=" ("字符串"), w429, " AND CODE_ID=" ("字符串"), w434) -> (w439:string)
                    n180 = call-poly <vilib>:"DB Tools Open Connection.vi"("error in (no error)"=w438, "connection information"=w437) -> ("error out"=w444:errorcluster, "connection reference"=w443:T14)  [unwired: 6 in]
                    n181 = call-poly <vilib>:"DB Tools Execute Query.vi"("error in (no error)"=w444, "SQL query"=w439, "connection reference"=w443) -> ("error out"=w441:errorcluster, "recordset reference"=w440:T18)  [unwired: 5 in]
                    n182 = call-poly <vilib>:"DB Tools Fetch Recordset Data.vi"("error in (no error)"=w441, "recordset reference"=w440) -> ("error out"=w445:errorcluster, "recordset data"=w442:variant[][])  [unwired: 3 in, 1 out]
                    n183 = Variant To Data(error in=w445, type=string[][] [], Variant=w442) -> (data=w446:string[][])  [unwired: 1 out]
                    n184 = Index Array(array=w446, index (row)=0 ("索引 (行)")) -> (element=w447:string[])  [unwired: 1 in]
                    n185 = Index Array(array=w447, index=0 ("索引 (行)")) -> (element=w435:string)
                    n186 = case shown="\"OK\"" w435 {
                      frame "假", Default {
                      }
                      frame "真" {
                      }
                      frame "OK" {
                        n187 = local read "产品条码"() -> (w448:string)
                        n188 = String Length(string=w448) -> (length=w452:i32)
                        n189 = Greater?(x=w452, y=1) -> (0:w453:bool)
                        n190 = case shown="真" w453 {
                          frame False {
                          }
                          frame True {
                            n191 = shared-variable "我的电脑\\A131258.lvlib\\当前曲线"(i16 1002 ("当前曲线")) -> ()  [unwired: 1 in, 1 out]
                          }
                        }
                        n192 = property on="上序结果" class="Bool (严格)"("Colors [4]"=cluster{u32, u32}[] [{6618880, 6618880}, {6618880, 6618880}, {6618880, 6618880}, {6618880, 6618880}]) -> ()  [unwired: 2 in, 2 out]
                        n193 = local write "字符串"("合格" ("字符串")) -> ()
                      }
                      frame "NG" {
                        n194 = property on="上序结果" class="Bool (严格)"("Colors [4]"=cluster{u32, u32}[] [{16711680, 16711680}, {16711680, 16711680}, {16711680, 16711680}, {16711680, 16711680}]) -> ()  [unwired: 2 in, 2 out]
                        n195 = shared-variable "我的电脑\\A131258.lvlib\\当前曲线"(i16 0 ("当前曲线")) -> ()  [unwired: 1 in, 1 out]
                        n196 = local write "字符串"("不合格" ("字符串")) -> ()
                      }
                      frame "" {
                        n197 = shared-variable "我的电脑\\A131258.lvlib\\当前曲线"(i16 0 ("当前曲线")) -> ()  [unwired: 1 in, 1 out]
                      }
                    }
                  }
                }
              }
            }
          }
        }
        n198 = control-ref of="振动判定范围"() -> (w33:refnum<vi>)
        n199 = call <vilib>:"Application Directory.vi"() -> ("Application Directory"=w35:path)
        n200 = control-ref of="振动判定"() -> (w32:refnum<vi>)
        n201 = Build Path(base path=w35, name or relative path="config\\Product_Parameter.ini" ("名称或相对路径")) -> (appended path=w31:path)
        n202 = Build Array(w33, w32) -> (w30:refnum<vi>[])
        n203 = event shown="[8] 前面板关闭？" {
          selector: _ -> [_ _ _ _ _ _ _ _ _ _ _ _ _]
          dyn-events: _ -> [_ _ _ _ _ _ _ _ _ _ _ _ _]
          timeout: 10 -> [_ _ _ _ _ _ _ _ _ _ _ _ _]
          tunnel: w31 -> [w38 w48 _ w95 w113 _ w125 _ _ _ _ _ _]
          tunnel: w30 -> [_ _ _ w94 w114 _ w124 _ _ _ _ _ _]
          event Timeout {
            n204 = event-data() -> ()  [unwired: 1 in, 3 out]
            n205 = call <vilib>:"Open Config Data.vi"("create file if necessary (T)"=TRUE, "configuration file path"=w38) -> ("error out"=w44:errorcluster, "refnum"=w43:T19)  [unwired: 7 in, 1 out]
            n206 = call <vilib>:"Get Section Names.vi"("error in (no error)"=w44, "refnum"=w43) -> ("error out"=w46:errorcluster, "section names"=w42:string[], "refnum out"=w45:T19)  [unwired: 7 in]
            n207 = control-ref of="请选择要删除的产品"() -> (w40:refnum<vi>)
            n208 = call <vilib>:"Close Config Data.vi"("error in (no error)"=w46, "refnum"=w45) -> ()  [unwired: 8 in, 2 out]
            n209 = control-ref of="产品型号"() -> (w41:refnum<vi>)
            n210 = property on="属性节点" class="CmbBox"(reference=w41, "Strings[]"=w42) -> ()  [unwired: 1 in, 2 out]
            n211 = property on="属性节点" class="CmbBox"(reference=w40, "Strings[]"=w42) -> ()  [unwired: 1 in, 2 out]
          }
          event "删除": Value Change {
            n212 = event-data() -> ("NewVal"=w47:bool)  [unwired: 1 in, 5 out]
            n213 = case shown="真" w47 {
              tunnel: w48 -> [_ w50]
              frame False {
              }
              frame True {
                n214 = Concatenate Strings("确认删除“", "请选择要删除的产品", "”吗？") -> (w52:string)
                n215 = Two Button Dialog(message=w52) -> (T button?=w51:bool)  [unwired: 2 in]
                n216 = case shown="真" w51 {
                  tunnel: w50 -> [_ w56]
                  tunnel: "请选择要删除的产品" -> [_ w55]
                  frame False {
                  }
                  frame True {
                    n217 = call <vilib>:"Open Config Data.vi"("configuration file path"=w56) -> ("error out"=w58:errorcluster, "refnum"=w61:T19)  [unwired: 8 in, 1 out]
                    n218 = call <vilib>:"Remove Section.vi"("section"=w55, "error in (no error)"=w58, "refnum"=w61) -> ("error out"=w60:errorcluster, "section exists?"=w57:bool, "refnum out"=w59:T19)  [unwired: 6 in]
                    n219 = call <vilib>:"Close Config Data.vi"("error in (no error)"=w60, "refnum"=w59) -> ()  [unwired: 8 in, 2 out]
                    n220 = case shown="假" w57 {
                      frame False {
                        n221 = One Button Dialog(message="删除失败！\n请确认产品存在！" ("消息")) -> ()  [unwired: 1 in, 1 out]
                      }
                      frame True {
                        n222 = One Button Dialog(message="删除成功！" ("消息")) -> ()  [unwired: 1 in, 1 out]
                      }
                    }
                  }
                }
              }
            }
          }
          event "确定": Value Change {
            n223 = event-data() -> ("NewVal"=w64:bool)  [unwired: 1 in, 5 out]
            n224 = case shown="真" w64 {
              frame False {
              }
              frame True {
                n225 = stacked-sequence {
                  frame #0 {
                    w66 = "参数装载成功！" ("消息")
                    n226 = shared-variable "我的电脑\\Global.lvlib\\产品型号"("产品型号") -> ()  [unwired: 1 in, 1 out]
                    n227 = call "浮动通知.vi"("通知内容"=w66) -> ()  [unwired: 11 in]
                    n228 = One Button Dialog(message=w66) -> ()  [unwired: 1 in, 1 out]
                    "产品型号" <- "产品型号"
                  }
                  frame #1 {
                    n229 = global read "Global2.vi" "联机模式"() -> (w67:enum16{"单机", "追溯"})
                    n230 = case shown="\"追溯\"" w67 {
                      frame "单机", Default {
                      }
                      frame "追溯" {
                        n231 = shared-variable "我的电脑\\Global.lvlib\\产品型号"() -> (w72:string)  [unwired: 1 in, 1 out]
                        n232 = call "Get_Device_ID.vi"() -> ("Device_ID"=w73:string)  [unwired: 10 in, 1 out]
                        n233 = local write "deviceID"(w73) -> ()
                        n234 = call "GET_PRODUCT_ID.vi"("PRODFUCT_NAME"=w72) -> ("PRODUCT_ID"=w68:string)  [unwired: 10 in]
                        n235 = call "查询前序设备.vi"("PRODUCT_ID"=w68) -> ("前序工位"=w69:string[])  [unwired: 10 in]
                        n236 = local write "productID"(w68) -> ()
                        n237 = Index Array(array=w69, index=0 ("索引")) -> (element=w70:string)
                        n238 = local write "FdeviceID"(w70) -> ()
                      }
                    }
                  }
                  frame #2 {
                    n239 = global read "Global2.vi" "联机模式"() -> (w74:enum16{"单机", "追溯"})
                    n240 = case shown="\"追溯\"" w74 {
                      tunnel: w74 -> [_ w78]
                      frame "单机", Default {
                      }
                      frame "追溯" {
                        n241 = local read "用户名"() -> (w76:string)
                        n242 = call "GetSQLstring.vi"("联机模式"=w78) -> ("错误输出"=w92:errorcluster, "连接字符串"=w93:string)  [unwired: 9 in]
                        n243 = call-poly <vilib>:"DB Tools Open Connection.vi"("error in (no error)"=w92, "connection information"=w93) -> ("error out"=w85:errorcluster, "connection reference"=w86:T14)  [unwired: 6 in]
                        n244 = Concatenate Strings("SELECT USER_ID FROM [User]  WHERE USER_NAME ='" ("字符串"), w76, "'" ("字符串")) -> (w91:string)
                        n245 = call-poly <vilib>:"DB Tools Execute Query.vi"("error in (no error)"=w85, "SQL query"=w91, "connection reference"=w86) -> ("error out"=w89:errorcluster, "recordset reference"=w90:T18)  [unwired: 5 in]
                        n246 = call-poly <vilib>:"DB Tools Fetch Recordset Data.vi"("error in (no error)"=w89, "recordset reference"=w90) -> ("error out"=w84:errorcluster, "recordset data"=w88:variant[][])  [unwired: 3 in, 1 out]
                        n247 = Variant To Data(error in=w84, type=string[][] [], Variant=w88) -> (data=w83:string[][])  [unwired: 1 out]
                        n248 = Index Array(array=w83, index (row)=0 ("索引 (行)")) -> (element=w81:string[])  [unwired: 1 in]
                        n249 = Index Array(array=w81, index=0 ("索引 (行)")) -> (element=w77:string)
                        n250 = local write "USERID"(w77) -> ()
                      }
                    }
                  }
                }
              }
            }
          }
          event "添加": Value Change {
            n251 = event-data() -> ("NewVal"=w96:bool)  [unwired: 1 in, 5 out]
            n252 = local read "请选择要删除的产品"() -> (w97:string)
            n253 = call <vilib>:"Trim Whitespace.vi"("string"=w97) -> ("trimmed string"=w98:string)  [unwired: 1 in]
            n254 = White Space?(1:w98) -> (0:w99:bool)
            n255 = case shown="假" w99 {
              tunnel: w94 -> [w102 _]
              tunnel: w96 -> [w101 _]
              tunnel: w95 -> [w100 _]
              frame False {
                n256 = case shown="真" w101 {
                  tunnel: w102 -> [_ w104]
                  tunnel: w100 -> [_ w103]
                  frame False {
                  }
                  frame True {
                    n257 = for {
                      tunnel: w104 -> [w107] mode=indexing
                      tunnel: w103 -> [w106]
                      n258 = call "Read_Write ParaINI File.vi"("Mode"=enum16{"Read", "Write"}."Write", "Section"="请输入添加的产品名称", "Filepath"=w106, "Ctl Refnum"=w107) -> ()  [unwired: 7 in, 1 out]
                    }
                  }
                }
              }
              frame True {
                w109 = 64 items=["None"=0, "Hand, Error, Stop"=16, "Question"=32, "Exclamation, Warning"=48, "Asterisk, Information"=64] ("icon")
                w110 = 0 items=["OK", "OKCancel", "AbortRetryIgnore", "YesNoCancel", "YesNo", "RetryCancel"] ("buttons")
                n259 = call "信息框（标题、文本、图标）.vi"("icon"=w109, "buttons"=w110, "caption"="添加失败", "text"="请输入产品名称!") -> ()  [unwired: 6 in, 2 out]
              }
            }
          }
          event "产品型号": Value Change {
            n260 = event-data() -> ()  [unwired: 1 in, 6 out]
            n261 = stacked-sequence {
              tunnel: w114 -> [_ w116]
              tunnel: w113 -> [_ w115]
              frame #0 {
              }
              frame #1 {
                n262 = for {
                  tunnel: w116 -> [w119] mode=indexing
                  tunnel: w115 -> [w118]
                  n263 = local read "产品型号"() -> (w117:string)
                  n264 = call "Read_Write ParaINI File.vi"("Mode"=enum16{"Read", "Write"}."Read", "Section"=w117, "Filepath"=w118, "Ctl Refnum"=w119) -> ()  [unwired: 7 in, 1 out]
                }
              }
            }
          }
          event "退出": Value Change {
            n265 = event-data() -> ()  [unwired: 1 in, 6 out]
            n266 = control-ref of="本VI"() -> (w123:refnum<vi>)
            n267 = invoke class="VI" method="FP.Close"(reference=w123) -> (reference out=w121:refnum<vi>, error out=w122:errorcluster)  [unwired: 2 in, 1 out]
            n268 = Close Reference(reference=w121, error in (no error)=w122) -> ()  [unwired: 1 out]
          }
          event "更新": Value Change {
            n269 = event-data() -> ("NewVal"=w126:bool)  [unwired: 1 in, 5 out]
            n270 = case shown="真" w126 {
              tunnel: w125 -> [_ w129]
              tunnel: w124 -> [_ w128]
              frame False {
              }
              frame True {
                n271 = for {
                  tunnel: w129 -> [w134]
                  tunnel: w128 -> [w133] mode=indexing
                  tunnel: [w132] -> w127
                  n272 = local read "产品型号"() -> (w136:string)
                  n273 = call "Read_Write ParaINI File.vi"("Mode"=enum16{"Read", "Write"}."Write", "Section"=w136, "Filepath"=w134, "Ctl Refnum"=w133) -> ("error out"=w132:errorcluster)  [unwired: 7 in]
                }
                n274 = case shown="无错误" w127 {
                  frame No Error {
                    n275 = call "浮动通知.vi"("通知内容"="更新成功！") -> ()  [unwired: 11 in]
                  }
                  frame Error {
                    n276 = call "浮动通知.vi"("通知内容"="更新失败！") -> ()  [unwired: 11 in]
                  }
                }
              }
            }
          }
          event "请输入添加的产品名称": Value Change {
            n277 = event-data() -> ("NewVal"=w138:string)  [unwired: 1 in, 5 out]
            n278 = control-ref of="产品型号"() -> (w137:refnum<vi>)
            n279 = property on="属性节点" class="CmbBox"(reference=w137) -> ("Strings[]"=w139:string[])  [unwired: 1 in, 2 out]
            n280 = for {
              tunnel: w138 -> [w140]
              tunnel: w139 -> [w141] mode=indexing
              n281 = Equal?(x=w140, y=w141) -> (x = y?=w142:bool)
              n282 = case shown="真" w142 {
                tunnel: w140 -> [_ w143]
                frame False {
                }
                frame True {
                  n283 = stacked-sequence {
                    tunnel: w143 -> [w149 _]
                    frame #0 {
                      w144 = 64 items=["None"=0, "Hand, Error, Stop"=16, "Question"=32, "Exclamation, Warning"=48, "Asterisk, Information"=64] ("icon")
                      w145 = 0 items=["OK", "OKCancel", "AbortRetryIgnore", "YesNoCancel", "YesNo", "RetryCancel"] ("buttons")
                      n284 = Concatenate Strings("已经存在产品”" ("text"), w149, "“\n请勿重复添加！" ("字符串")) -> (w147:string)
                      n285 = call "信息框（标题、文本、图标）.vi"("icon"=w144, "buttons"=w145, "caption"="产品重复", "text"=w147) -> ()  [unwired: 6 in, 2 out]
                    }
                    frame #1 {
                      n286 = local write "请输入添加的产品名称"("" ("请输入添加的产品名称")) -> ()
                    }
                  }
                }
              }
            }
          }
          event Panel Close? {
            n287 = event-data() -> ()  [unwired: 1 in, 4 out]
            n288 = control-ref of="本VI"() -> (w152:refnum<vi>)
            n289 = vi-ref "传感器读取.vi"() -> (w155:refnum<vi>)
            n290 = global write "Global.vi" "程序关闭"(TRUE ("程序关闭")) -> ()
            n291 = invoke class="VI" method="FP.Close"(reference=w152) -> (reference out=w153:refnum<vi>, error out=w154:errorcluster)  [unwired: 2 in, 1 out]
            n292 = invoke class="VI" method="FP.Close"(reference=w155) -> (reference out=w156:refnum<vi>, error out=w157:errorcluster)  [unwired: 2 in, 1 out]
            n293 = Close Reference(reference=w153, error in (no error)=w154) -> ()  [unwired: 1 out]
            n294 = Close Reference(reference=w156, error in (no error)=w157) -> ()  [unwired: 1 out]
            n295 = event-data("Discard?"=TRUE ("放弃？")) -> ()  [unwired: 1 in, 1 out]
          }
          event "确定按钮": Value Change {
            n296 = event-data() -> ()  [unwired: 1 in, 6 out]
            n297 = vi-ref "User_manager.vi"() -> (w161:refnum<vi>)
            n298 = call "CallVI.vi"("VI引用"=w161, "状态"=T4."Maximized") -> ()  [unwired: 11 in, 3 out]
          }
          event "设备故障": Value Change {
            n299 = event-data() -> ()  [unwired: 1 in, 6 out]
            n300 = global read "Global2.vi" "用户信息"() -> (w167:T5)
            n301 = Unbundle By Name(w167) -> ("用户名"=w165:string)
            n302 = Bundle("设备名称"="芯轴分总成NVH", "用户名"=w165, "设备状态"="设备状态", "附加信息"="附加信息") -> (w162:T20)  [unwired: 1 in]
            n303 = vi-ref "client.vi"() -> (w169:refnum<vi>)
            n304 = invoke class="VI" method="Ctrl Val.Set"(reference=w169, "Control Name"="设备信息" ("控件名"), "Value"=w162) -> ()  [unwired: 2 in, 5 out]
          }
          event "设备缺料": Value Change {
            n305 = event-data() -> ()  [unwired: 1 in, 6 out]
            n306 = global read "Global2.vi" "用户信息"() -> (w175:T5)
            n307 = Unbundle By Name(w175) -> ("用户名"=w173:string)
            n308 = Bundle("设备名称"="芯轴分总成NVH", "用户名"=w173, "设备状态 2"="设备状态 2", "附加信息 2"="附加信息 2") -> (w170:T21)  [unwired: 1 in]
            n309 = vi-ref "client.vi"() -> (w177:refnum<vi>)
            n310 = invoke class="VI" method="Ctrl Val.Set"(reference=w177, "Control Name"="设备信息" ("控件名"), "Value"=w170) -> ()  [unwired: 2 in, 5 out]
          }
          event "质量报警": Value Change {
            n311 = event-data() -> ()  [unwired: 1 in, 6 out]
            n312 = global read "Global2.vi" "用户信息"() -> (w183:T5)
            n313 = Unbundle By Name(w183) -> ("用户名"=w181:string)
            n314 = Bundle("设备名称"="芯轴分总成NVH", "用户名"=w181, "设备状态 3"="设备状态 3", "附加信息 3"="附加信息 3") -> (w178:T22)  [unwired: 1 in]
            n315 = vi-ref "client.vi"() -> (w185:refnum<vi>)
            n316 = invoke class="VI" method="Ctrl Val.Set"(reference=w185, "Control Name"="设备信息" ("控件名"), "Value"=w178) -> ()  [unwired: 2 in, 5 out]
          }
        }
        n317 = global read "Global.vi" "程序关闭"() -> (w29:bool)
      }
    }
  }
  n318 = call <userlib>:"Fit VI window to Largest Dec__ogtk.vi"("border spacing (2 px)"=0) -> ()  [unwired: 5 in, 2 out]
